vi "PH_Sixpack_Switch.PC Set Direction.vi"(0 "i ref in":refnum<vi>, 2 "Direction":T1, 5 "error IO":errorcluster) -> (14 "i ref out":refnum<vi>, 19 "error out":errorcluster)   [LabVIEW 2014, in "PH_Sixpack_Switch.lvlib"]
doc: "This is the Proc Case of \"set Direction\"."
uses:
  PH_Sixpack_Switch.lvlib
  PH_Basics/PH_Stepmotor_BaseClass/PH_Stepmotor_BaseClass.Axis Direction.ctl
  PH_Basics/PH_AxisGUI_BaseClass/PH_AxisGUI_BaseClass.lvlib
  PH_Basics/PH_Stepmotor_BaseClass/PH_Stepmotor_BaseClass.lvlib
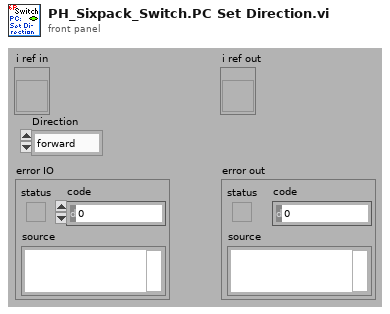
[diagram p1: front panel]
types:
  T1 = typedef "PH_Stepmotor_BaseClass.lvlib/PH_Stepmotor_BaseClass.Axis Direction.ctl" = enum16{"forward", "backward"}
  T2 = typedef "PH_Sixpack_Switch.lvlib/PH_Sixpack_Switch.i attribute.ctl" = cluster{"GUI Refs":cluster{"Delete":refnum<vi>, "Move":refnum<vi>, "Direction":refnum<vi>}, "remote controlled?":bool, "Move":bool, "Direction":T1}
  T3 = typedef "PH_AxisGUI_BaseClass.lvlib/PH_AxisGUI_BaseClass.i attribute.ctl" = cluster{"Axes":T4[]}
  T4 = typedef "PH_AxisGUI_BaseClass.lvlib/PH_AxisGUI_BaseClass.Axis Attributes.ctl" = cluster{"Axis GUI Refs":T5, "Address":T6, "Name":string, "Label \"Back\"":string, "Labell \"Forth\"":string, "Moving?":bool}
  T5 = typedef "PH_AxisGUI_BaseClass.lvlib/PH_AxisGUI_BaseClass.Axis GUI Refs.ctl" = cluster{"Back":refnum<vi>, "Forth":refnum<vi>, "Status":refnum<vi>, "Target":refnum<vi>, "Address":refnum<vi>, "Status Bar":refnum<vi>, "Settings":refnum<vi>, "Activity":refnum<vi>, "Clear Error":refnum<vi>}
  T6 = typedef "PH_Stepmotor_BaseClass.lvlib/PH_Stepmotor_BaseClass.Axis Address.ctl" = cluster{"Instance":string, "Motor Nr":i32}
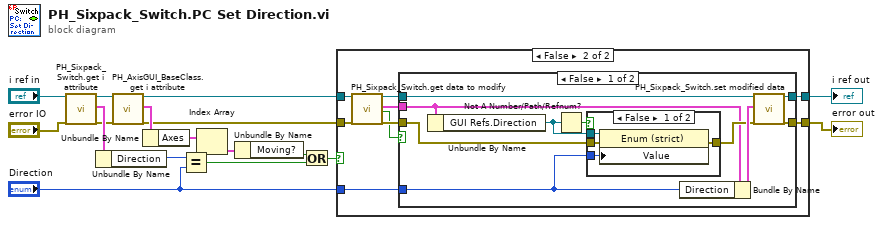
[diagram p0: block diagram]
diagram:
  n1 = call "PH_Sixpack_Switch.get i attribute.vi"("i ref in"="i ref in", "error in (no error)"="error IO") -> ("i ref out"=w9:refnum<vi>, "i attribute"=w17:T2, "error out"=w6:errorcluster)  [unwired: 15 in]
  n2 = Unbundle By Name(w17) -> ("Direction"=w5:T1)
  n3 = call "PH_AxisGUI_BaseClass.get i attribute.vi"("i ref in"=w9, "error in (no error)"=w6) -> ("i ref out"=w10:refnum<vi>, "i attribute"=w15:T3, "error out"=w11:errorcluster)  [unwired: 15 in]
  n4 = Unbundle By Name(w15) -> ("Axes"=w14:T4[])
  n5 = Equal?(x=w5, y="Direction") -> (x = y?=w1:bool)
  n6 = Index Array(array=w14) -> (element=w13:T4)  [unwired: 1 in]
  n7 = Unbundle By Name(w13) -> ("Moving?"=w2:bool)
  n8 = Or(x=w2, y=w1) -> (x .or. y?=w3:bool)
  n9 = case shown="False" w3 {
    tunnel: [w19 w27] -> w16
    tunnel: [w18 w25] -> w12
    tunnel: w10 -> [w19 w24]
    tunnel: w11 -> [w18 w23]
    tunnel: "Direction" -> [_ w20]
    frame True {
    }
    frame False {
      n10 = call "PH_Sixpack_Switch.get data to modify.vi"("i ref in"=w24, "error in (no error)"=w23) -> ("i ref out"=w28:refnum<vi>, "i attribute"=w21:T2, "timed out"=w22:bool, "error out"=w26:errorcluster)  [unwired: 14 in]
      n11 = case shown="False" w22 {
        tunnel: w28 -> [w38 w45]
        tunnel: [w37 w45] -> w27
        tunnel: w26 -> [w32 w44]
        tunnel: [w36 w44] -> w25
        tunnel: w21 -> [w33 _]
        tunnel: w20 -> [w31 _]
        frame False {
          n12 = Unbundle By Name(w33) -> ("GUI Refs.Direction"=w30:refnum<vi>)
          n13 = Not A Number/Path/Refnum?(number/path/refnum=w30) -> (NaN/Path/Refnum?=w29:bool)
          n14 = case shown="False" w29 {
            tunnel: [w42 w43] -> w34
            tunnel: w32 -> [w41 w43]
            tunnel: w30 -> [w40 _]
            tunnel: w31 -> [w39 _]
            frame False {
              n15 = property class="Enum (strict)"(reference=w40, error in=w41, "Value"=w39) -> (error out=w42:errorcluster)  [unwired: 1 out]
            }
            frame True {
            }
          }
          n16 = Bundle By Name(cluster=w33, "Direction"=w31) -> (w35:T2)
          n17 = call "PH_Sixpack_Switch.set modified data.vi"("i ref in"=w38, "i attribute"=w35, "error in (no error)"=w34) -> ("i ref out"=w37:refnum<vi>, "error out"=w36:errorcluster)  [unwired: 15 in]
        }
        frame True {
        }
      }
    }
  }
  "error out" <- w12
  "i ref out" <- w16
